vi "Digital IO.vi"(8 "error in (no error)":errorcluster, 10 "Refnum In2":refnum<k21>, 11 "Refnum in":refnum<k21>) -> (0 "error out":errorcluster, 1 "cluster":T1, 2 "task out 2":refnum<k21>, 3 "task out":refnum<k21>, 4 "cluster 2":T2)   [LabVIEW 2017]
uses:
  <vilib>/DAQmx/read.llb/DAQmx Read (Digital 1D Bool NChan 1Samp 1Line).vi
  <vilib>/DAQmx/miscellaneous.llb/DAQmx Fill In Error Info.vi
  GV/MachineStatusGV.vi
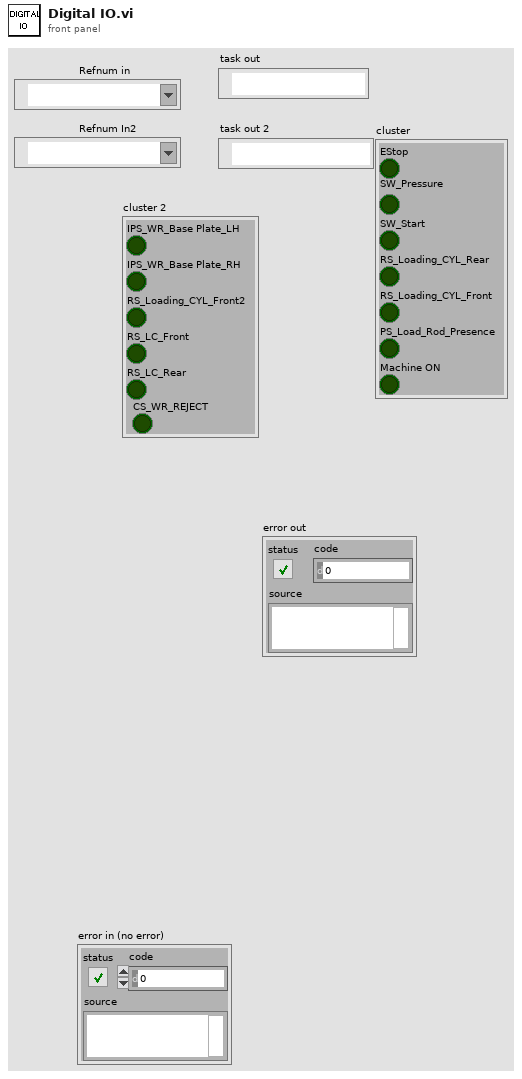
[diagram p1: front panel]
types:
  T1 = cluster{"EStop":bool, "SW_Pressure":bool, "SW_Start":bool, "RS_Loading_CYL_Rear":bool, "RS_Loading_CYL_Front":bool, "PS_Load_Rod_Presence":bool, "Machine ON":bool}
  T2 = cluster{"IPS_WR_Base Plate_LH":bool, "IPS_WR_Base Plate_RH":bool, "RS_Loading_CYL_Front2":bool, "RS_LC_Front":bool, "RS_LC_Rear":bool, "CS_WR_REJECT":bool}
  T3 = cluster{"data[0]":bool, "data[1]":bool, "data[2]":bool, "data[3]":bool, "data[4]":bool, "data[5]":bool}
  T4 = cluster{"data[0]":bool, "data[1]":bool, "data[2]":bool, "data[3]":bool, "data[4]":bool, "data[5]":bool, "data[6]":bool}
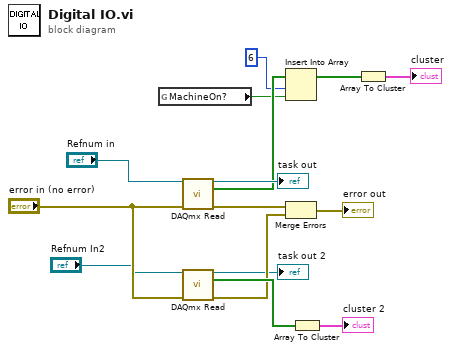
[diagram p0: block diagram]
diagram:
  n1 = global read "MachineStatusGV.vi" "MachineOn?"() -> (w6:bool)
  n2 = call-poly <vilib>:"DAQmx Read.vi"("task/channels in"="Refnum in", "error in"="error in (no error)") -> ("task out"=→"task out":refnum<k21>, "data"=w7:bool[], "error out"=w13:errorcluster)  [unwired: 11 in]
  n3 = call-poly <vilib>:"DAQmx Read.vi"("task/channels in"="Refnum In2", "error in"="error in (no error)") -> ("task out"=→"task out 2":refnum<k21>, "data"=w14:bool[], "error out"=w12:errorcluster)  [unwired: 11 in]
  n4 = Insert Into Array(array=w7, index=6, new element=w6) -> (w4:bool[])
  n5 = Merge Errors(w13, w12) -> (→"error out":errorcluster)
  n6 = Array To Cluster(array=w14) -> (cluster=→"cluster 2":T3)
  n7 = Array To Cluster(array=w4) -> (cluster=→"cluster":T4)
